vi "CSM - Run Script - Advance.vi"(0 "CSM Scripts":string, 1 "Current Module (\"\" to Generate an ID)":string, 7 "Continue If Error? (F)":bool, 9 "Wait (5000ms)":i32=5000, 11 "error in (no error)":errorcluster, 12 "Response Timeout (-2 Using Global Settings)":i32=-2) -> (4 "Response":string[](array[string]), 10 "Scripts Left":string, 15 "error out":errorcluster)   [LabVIEW 2020]
doc: "Executes multiple CSM commands in a single batch, supporting synchronous messages, asynchronous messages, and registrations.\n\n\n> [!NOTE] <b>CSM Message Target Module Description</b>\n>\n> In Normal Mode, the target module for a CSM message is the specified module name.\n> System-level modules start with a `.` in their name. The target module for a CSM message includes the `.` in the name. For example, if the requested module name is `.System`, the target module for the CSM message is `.System`.\n> In Worker Mode, the target module for a CSM message can only be the overall module name, not the node name. For example, if the requested module name is `Worker#`, the target module for the CSM message is `Worker`.\n> In Chain of Responsibility Mode, the target module for a CSM message can only be the overall module name, not the node name. For example, if the requested module name is `Chain$1`, the target module for the CSM message is `Chain`.\n\n\n-- <b>Controls</b> --\n- <b>Current Module (\"\" to Generate an ID)</b>: Name of the current module. If empty, a temporary ID is generated for debugging purposes to identify the location.\n- <b>CSM Scripts</b>: CSM commands to execute.\n- <b>Continue If Error? (F)</b>: Whether to continue execution if an error occurs. The default is FALSE, which specifies to not continue.\n- <b>Wait (5000 ms)</b>: Timeout duration for waiting module to be alive. The default is 5000 ms.\n- <b>Response Timeout (-2 Using Global Settings)</b>: Timeout for synchronous calls. The default is -2, which uses the global setting. You can set the global timeout using the CSM - Set TMO of Sync-Reply VI.\n\n-- <b>Indicators</b> --\n- <b>Response</b>: Returned results from executing the script. Only synchronous messages carry returns. The corresponding column for other commands will be an empty string.\n- <b>Scripts Left</b>: Remaining unexecuted scripts."
uses:
  <userlib>/_NEVSTOP/Communicable State Machine(CSM)/AdvanceAPI/CSM - Broadcast Message Type.ctl
  <userlib>/_NEVSTOP/Communicable State Machine(CSM)/Communicable State Machine.lvlib
  <userlib>/_NEVSTOP/Communicable State Machine(CSM)/_Shared/CSM Shared.lvlib
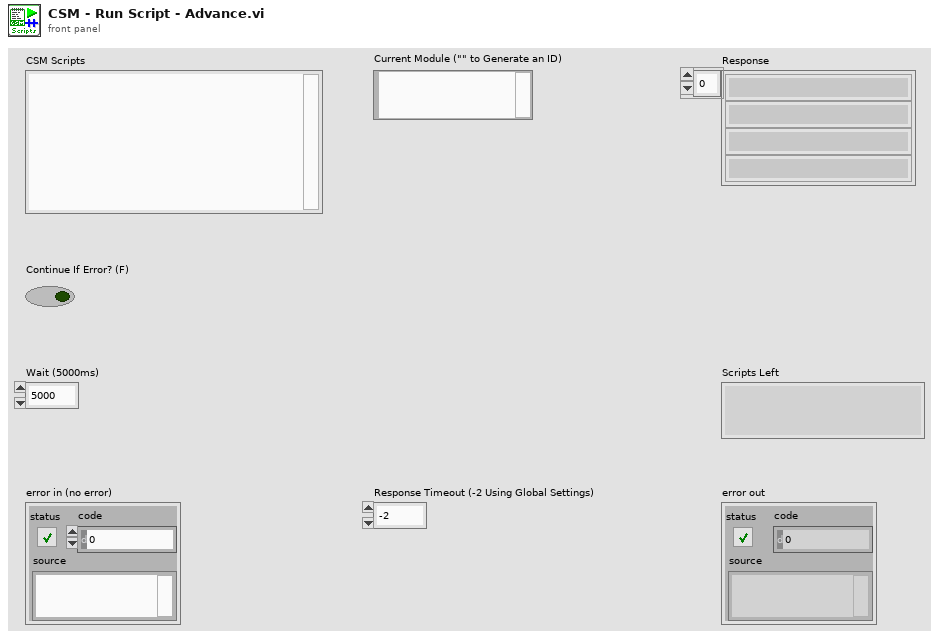
[diagram p1: front panel]
types:
  T1 = typedef "Communicable State Machine.lvlib/CSM - Broadcast Message Type.ctl" = enum16{"<Null>", "Status", "Interrupt"}
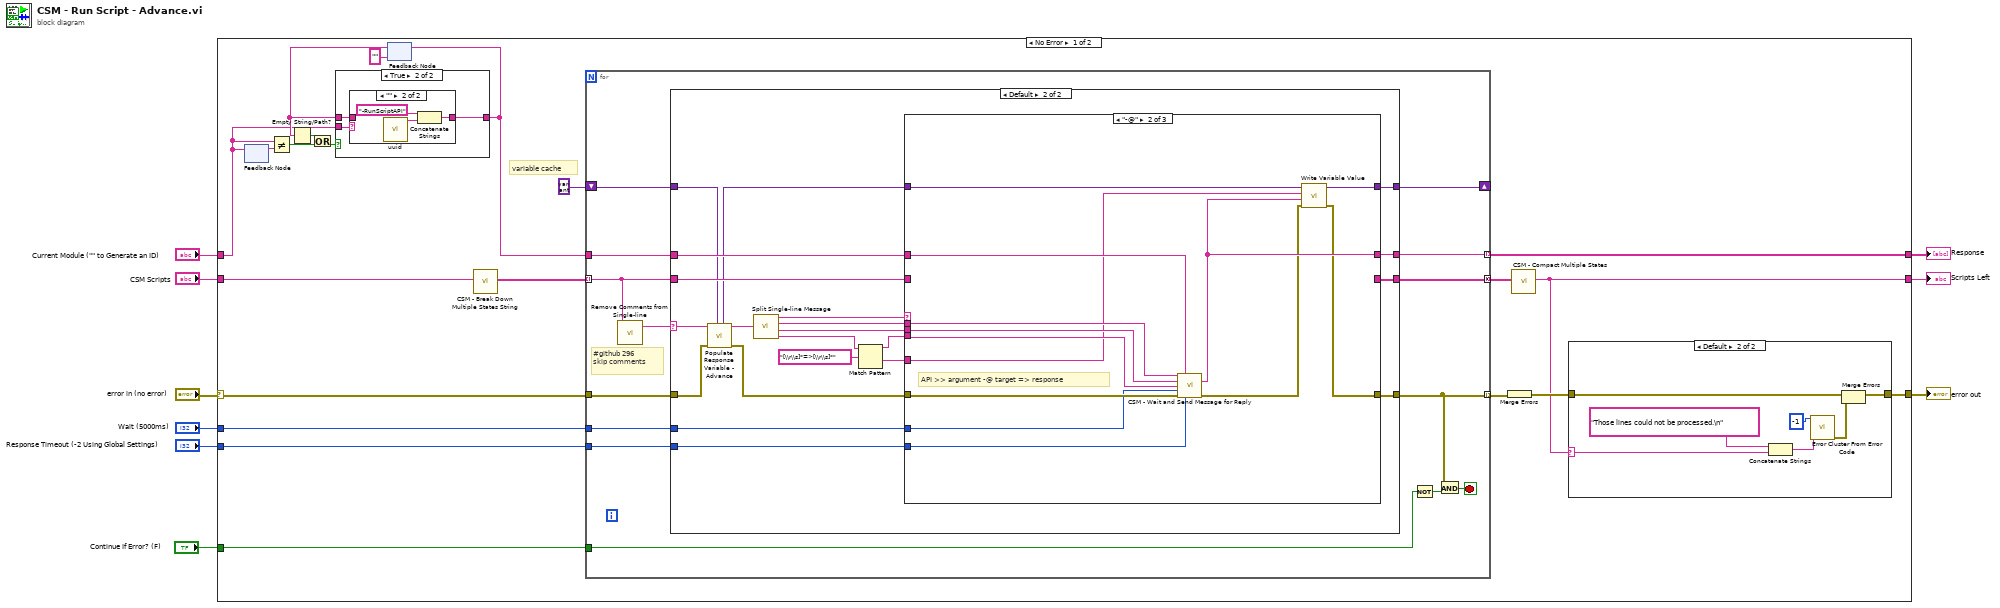
[diagram p0: block diagram]
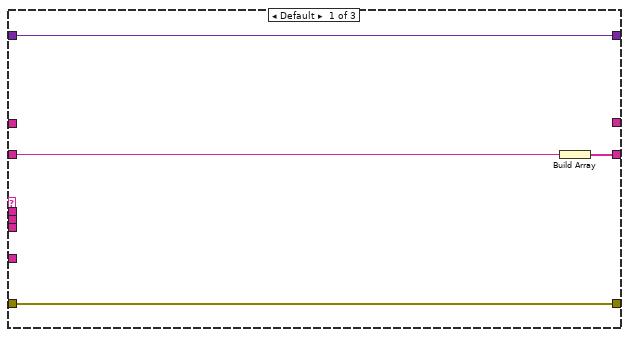
[diagram p4: hidden frame]
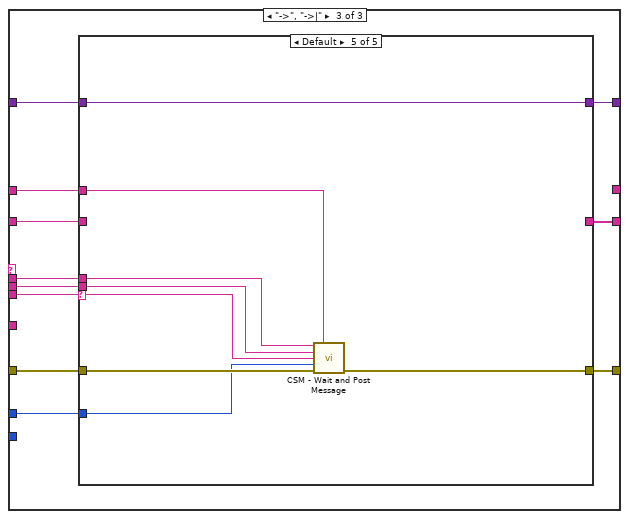
[diagram p5: hidden frame]
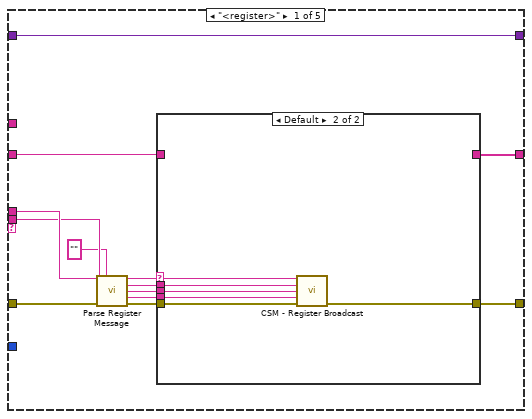
[diagram p6: hidden frame]
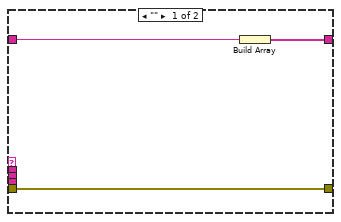
[diagram p7: hidden frame]
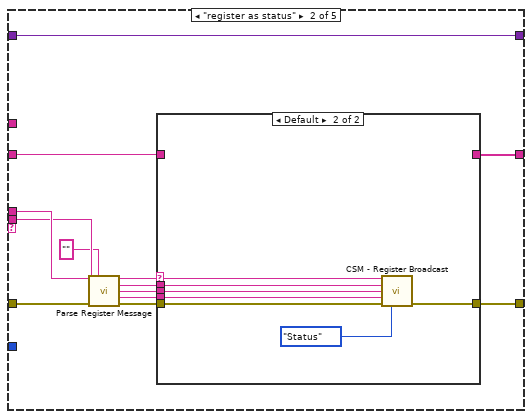
[diagram p8: hidden frame]
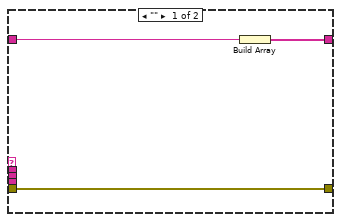
[diagram p9: hidden frame]
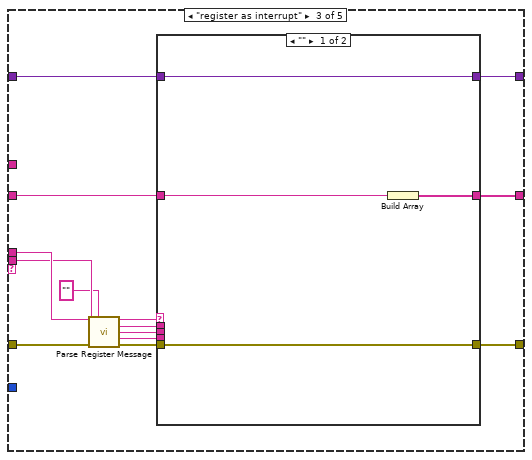
[diagram p10: hidden frame]
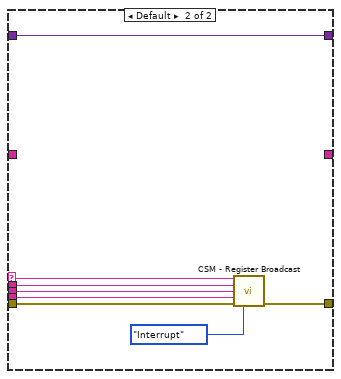
[diagram p11: hidden frame]
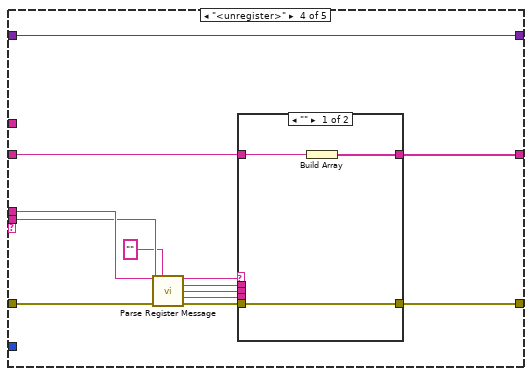
[diagram p12: hidden frame]
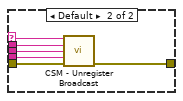
[diagram p13: hidden frame]
diagram:
  n1 = case shown="No Error" "error in (no error)" {
    selector: "error in (no error)" -> [w28 w209]
    tunnel: "CSM Scripts" -> [w27 _]
    tunnel: [w24 _] -> w7
    tunnel: [w23 w209] -> w6
    tunnel: "Current Module (\"\" to Generate an ID)" -> [w12 _]
    tunnel: "Response Timeout (-2 Using Global Settings)" -> [w22 _]
    tunnel: "Wait (5000ms)" -> [w21 _]
    tunnel: "Continue If Error? (F)" -> [w20 _]
    tunnel: [w19 _] -> w1
    frame No Error {
      # "variable cache"
      n2 = feedback #1() -> (w18:string)  [unwired: 1 in]
      n3 = feedback-in #1(w12) -> ()
      n4 = Not Equal?(x=w12, y=w18) -> (x != y?=w17:bool)
      n5 = feedback #2("") -> (w14:string)
      n6 = Empty String/Path?(string/path=w14) -> (empty?=w13:bool)
      n7 = Or(x=w13, y=w17) -> (x .or. y?=w15:bool)
      n8 = case shown="True" w15 {
        tunnel: w14 -> [w201 w204]
        tunnel: w12 -> [_ w203]
        tunnel: [w201 w202] -> w11
        frame False {
        }
        frame True {
          n9 = case shown="\"\"" w203 {
            selector: w203 -> [w205 _]
            tunnel: [w205 w206] -> w202
            tunnel: w204 -> [_ _]
            frame Default {
            }
            frame "" {
              n10 = call <userlib>:"uuid.vi"() -> ("UUID"=w207:string)  [unwired: 11 in]
              n11 = Concatenate Strings("-RunScriptAPI" ("Name (\"\" to Use UUID)"), w207) -> (w206:string)
            }
          }
        }
      }
      n12 = feedback-in #2(w11) -> ()
      n13 = call <userlib>:"CSM - Break Down Multiple States String.vi"("States"=w27) -> ("Multiple States"=w26:string[])  [unwired: 10 in]
      n14 = for {
        tunnel: w26 -> [w49] mode=indexing
        tunnel: w28 -> [w52]
        tunnel: [w44] -> w29 mode=indexing
        tunnel: [w50] -> w25 mode=concatenating
        tunnel: w11 -> [w48]
        tunnel: w22 -> [w47]
        tunnel: w21 -> [w46]
        tunnel: w20 -> [w43]
        tunnel: [w41] -> w19 mode=indexing
        shift-right: [w39] -> _
        shift-left: variant -> [w40]
        stop <- w45 stop-if-true
        # "#github 296\nskip comments"
        n15 = call <userlib>:"Remove Comments from Single-line.vi"("single-line text"=w49) -> ("single-line text without comments"=w51:string)  [unwired: 2 in]
        n16 = case shown="Default" w51 {
          selector: w51 -> [_ w62]
          tunnel: [w54 w75] -> w44
          tunnel: w52 -> [w54 w60]
          tunnel: [_ w71] -> w50
          tunnel: w49 -> [_ w70]
          tunnel: w48 -> [_ w69]
          tunnel: w47 -> [_ w68]
          tunnel: w46 -> [_ w67]
          tunnel: [_ w66] -> w41
          tunnel: w40 -> [w53 w64]
          tunnel: [w53 w65] -> w39
          frame "" {
          }
          frame Default {
            n17 = call "Populate Response Variable - Advance.vi"("Variant"=w64, "Error in"=w60, "String might with variables"=w62) -> ("Error out"=w59:errorcluster, "String out"=w61:string, "Variant Out"=w63:variant)  [unwired: 4 in]
            n18 = call <userlib>:"Split Single-line Message.vi"("single-line text"=w61) -> ("operator"=w74:string, "state"=w72:string, "args"=w73:string, "source/target"=w57:string)  [unwired: 6 in]
            n19 = Match Pattern(string=w57, regular expression="[\\r\\s]*=>[\\r\\s]*") -> (before substring=w56:string, after substring=w55:string)  [unwired: 1 in, 2 out]
            n20 = case shown="\"-@\"" w74 {
              tunnel: w56 -> [_ w81 w103]
              tunnel: w73 -> [_ w92 w102]
              tunnel: w72 -> [_ w91 w101]
              tunnel: w59 -> [w79 w90 w100]
              tunnel: [w79 w82 w99] -> w75
              tunnel: [w78 _ w98] -> w71
              tunnel: w70 -> [w77 _ w97]
              tunnel: w69 -> [_ w89 w96]
              tunnel: w68 -> [_ w88 _]
              tunnel: w67 -> [_ w87 w95]
              tunnel: [_ w84 _] -> w66
              tunnel: [w76 w85 w94] -> w65
              tunnel: w63 -> [w76 w86 w93]
              tunnel: w55 -> [_ w80 _]
              frame Default {
                n21 = Build Array(w77) -> (w78:string[])
              }
              frame "-@" {
                # "API >> argument -@ target => response"
                n22 = call <userlib>:"CSM - Wait and Send Message for Reply.vi"("State"=w91, "Current Module (\"\" to Generate an ID)"=w89, "Arguments (\"\")"=w92, "Target Module"=w81, "Wait (5000ms)"=w87, "Error In (No Error)"=w90, "Response Timeout (-2 Using Global Settings)"=w88) -> ("Response"=w84:string, "error out"=w83:errorcluster)  [unwired: 5 in, 2 out]
                n23 = call "Write Variable Value.vi"("Error in"=w83, "Response"=w84, "source/target"=w80, "Variant Out in"=w86) -> ("Error out"=w82:errorcluster, "Variant Out out"=w85:variant)  [unwired: 6 in]
              }
              frame "->", "->|" {
                n24 = case shown="Default" w103 {
                  selector: w103 -> [_ _ _ _ w200]
                  tunnel: w102 -> [w110 w131 w154 w178 w199]
                  tunnel: w101 -> [w111 w132 w155 w179 w198]
                  tunnel: w100 -> [w109 w130 w153 w177 w197]
                  tunnel: [w108 w129 w152 w176 w196] -> w99
                  tunnel: [w106 w127 w150 w174 _] -> w98
                  tunnel: w97 -> [w105 w126 w149 w173 _]
                  tunnel: w96 -> [_ _ _ _ w195]
                  tunnel: w95 -> [_ _ _ _ w194]
                  tunnel: [w104 w125 w148 w172 w193] -> w94
                  tunnel: w93 -> [w104 w125 w147 w172 w193]
                  frame "<register>" {
                    n25 = call <userlib>:"Parse Register Message.vi"("State"=w111, "Module Name"="", "Args"=w110) -> ("Target"=w115:string, "Source"=w114:string, "Status"=w113:string, "Api"=w112:string)  [unwired: 8 in, 1 out]
                    n26 = case shown="Default" w115 {
                      selector: w115 -> [_ w124]
                      tunnel: w114 -> [_ w123]
                      tunnel: w113 -> [_ w122]
                      tunnel: w112 -> [_ w121]
                      tunnel: w109 -> [w118 w120]
                      tunnel: [w118 w119] -> w108
                      tunnel: [w116 _] -> w106
                      tunnel: w105 -> [w117 _]
                      frame "" {
                        n27 = Build Array(w117) -> (w116:string[])
                      }
                      frame Default {
                        n28 = call <userlib>:"CSM - Register Broadcast.vi"("CSM Name(Empty for Broadcast Event)"=w124, "Source CSM Name (* as Default)"=w123, "Trigger"=w122, "API (If \"\", Same as Trigger)"=w121, "Error In"=w120) -> ("error out"=w119:errorcluster)  [unwired: 9 in, 1 out]
                      }
                    }
                  }
                  frame "register as status" {
                    n29 = call <userlib>:"Parse Register Message.vi"("State"=w132, "Module Name"="", "Args"=w131) -> ("Target"=w136:string, "Source"=w135:string, "Status"=w134:string, "Api"=w133:string)  [unwired: 8 in, 1 out]
                    n30 = case shown="Default" w136 {
                      selector: w136 -> [_ w146]
                      tunnel: w135 -> [_ w145]
                      tunnel: w134 -> [_ w144]
                      tunnel: w133 -> [_ w143]
                      tunnel: w130 -> [w139 w142]
                      tunnel: [w139 w141] -> w129
                      tunnel: [w137 _] -> w127
                      tunnel: w126 -> [w138 _]
                      frame "" {
                        n31 = Build Array(w138) -> (w137:string[])
                      }
                      frame Default {
                        n32 = call <userlib>:"CSM - Register Broadcast.vi"("CSM Name(Empty for Broadcast Event)"=w146, "Source CSM Name (* as Default)"=w145, "Trigger"=w144, "API (If \"\", Same as Trigger)"=w143, "Error In"=w142, "Priority (No Change)"=CSM_-_Broadcast_Message_Type."Status") -> ("error out"=w141:errorcluster)  [unwired: 8 in, 1 out]
                      }
                    }
                  }
                  frame "register as interrupt" {
                    n33 = call <userlib>:"Parse Register Message.vi"("State"=w155, "Module Name"="", "Args"=w154) -> ("Target"=w159:string, "Source"=w158:string, "Status"=w157:string, "Api"=w156:string)  [unwired: 8 in, 1 out]
                    n34 = case shown="\"\"" w159 {
                      selector: w159 -> [_ w171]
                      tunnel: w158 -> [_ w170]
                      tunnel: w157 -> [_ w169]
                      tunnel: w156 -> [_ w168]
                      tunnel: w153 -> [w163 w167]
                      tunnel: [w163 w166] -> w152
                      tunnel: [w161 _] -> w150
                      tunnel: w149 -> [w162 _]
                      tunnel: [w160 w164] -> w148
                      tunnel: w147 -> [w160 w164]
                      frame "" {
                        n35 = Build Array(w162) -> (w161:string[])
                      }
                      frame Default {
                        n36 = call <userlib>:"CSM - Register Broadcast.vi"("CSM Name(Empty for Broadcast Event)"=w171, "Source CSM Name (* as Default)"=w170, "Trigger"=w169, "API (If \"\", Same as Trigger)"=w168, "Error In"=w167, "Priority (No Change)"=CSM_-_Broadcast_Message_Type."Interrupt") -> ("error out"=w166:errorcluster)  [unwired: 8 in, 1 out]
                      }
                    }
                  }
                  frame "<unregister>" {
                    n37 = call <userlib>:"Parse Register Message.vi"("State"=w179, "Module Name"="", "Args"=w178) -> ("Target"=w183:string, "Source"=w182:string, "Status"=w181:string, "Api"=w180:string)  [unwired: 8 in, 1 out]
                    n38 = case shown="\"\"" w183 {
                      selector: w183 -> [_ w192]
                      tunnel: w182 -> [_ w191]
                      tunnel: w181 -> [_ w190]
                      tunnel: w180 -> [_ w189]
                      tunnel: w177 -> [w186 w188]
                      tunnel: [w186 w187] -> w176
                      tunnel: [w184 _] -> w174
                      tunnel: w173 -> [w185 _]
                      frame "" {
                        n39 = Build Array(w185) -> (w184:string[])
                      }
                      frame Default {
                        n40 = call <userlib>:"CSM - Unregister Broadcast.vi"("CSM Name(Empty for Broadcast Event)"=w192, "Source CSM Name (* as Default)"=w191, "Trigger"=w190, "API (\"*\" as Default)"=w189, "Error In"=w188) -> ("error out"=w187:errorcluster)  [unwired: 9 in, 1 out]
                      }
                    }
                  }
                  frame Default {
                    n41 = call <userlib>:"CSM - Wait and Post Message.vi"("State"=w198, "Current Module (\"\" to Generate an ID)"=w195, "Arguments (\"\")"=w199, "Target Module"=w200, "Wait (5000ms)"=w194, "Error In (No Error)"=w197) -> ("error out"=w196:errorcluster)  [unwired: 8 in, 1 out]
                  }
                }
              }
            }
          }
        }
        n42 = Not(x=w43) -> (.not. x?=w42:bool)
        n43 = And(x=w44, y=w42) -> (x .and. y?=w45:bool)
      }
      n44 = Merge Errors(w29) -> (w30:errorcluster)
      n45 = call <userlib>:"CSM - Compact Multiple States.vi"("Multiple States"=w25) -> ("States"=w24:string)  [unwired: 9 in]
      n46 = case shown="Default" w24 {
        selector: w24 -> [_ w34]
        tunnel: w30 -> [w31 w38]
        tunnel: [w31 w33] -> w23
        frame "" {
        }
        frame Default {
          n47 = Concatenate Strings("Those lines could not be processed.\n" ("String to Prepend to source (\"\")"), w34) -> (w35:string)
          n48 = call <vilib>:"Error Cluster From Error Code.vi"("error message (\"\")"=w35, "error code (0)"=-1 ("code")) -> ("error out"=w32:errorcluster)  [unwired: 7 in]
          n49 = Merge Errors(w38, w32) -> (w33:errorcluster)
        }
      }
    }
    frame Error {
    }
  }
  "error out" <- w6
  "Scripts Left" <- w7
  "Response" <- w1
